vi "CRYGet Next Color.vi"(11 "Type":enum16{"Curves", "Values", "Results", "WFM"}(ring)) -> (3 "Color":u32)   [LabVIEW 2013]
uses:
  Global/CRYCurve Library Global.vi
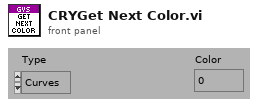
[diagram p1: front panel]
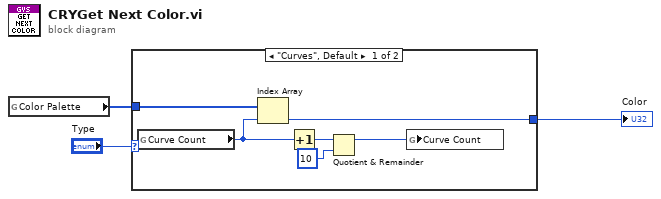
[diagram p0: block diagram]
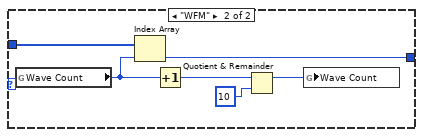
[diagram p2: hidden frame]
diagram:
  n1 = global read "CRYCurve Library Global.vi" "Color Palette"() -> (w2:u32[])
  n2 = case shown="\"Curves\", Default" "Type" {
    tunnel: w2 -> [w9 w15]
    tunnel: [w8 w14] -> w1
    frame "Curves", Default {
      n3 = global read "CRYCurve Library Global.vi" "Curve Count"() -> (w7:i32)
      n4 = Index Array(array=w9, index=w7) -> (element=w8:u32)
      n5 = Increment(x=w7) -> (x+1=w6:i32)
      n6 = Quotient & Remainder(x=w6, y=10) -> (x-y*floor(x/y)=w4:i32)  [unwired: 1 out]
      n7 = global write "CRYCurve Library Global.vi" "Curve Count"(w4) -> ()
    }
    frame "WFM" {
      n8 = global read "CRYCurve Library Global.vi" "Wave Count"() -> (w13:i32)
      n9 = Index Array(array=w15, index=w13) -> (element=w14:u32)
      n10 = Increment(x=w13) -> (x+1=w11:i32)
      n11 = Quotient & Remainder(x=w11, y=10) -> (x-y*floor(x/y)=w10:i32)  [unwired: 1 out]
      n12 = global write "CRYCurve Library Global.vi" "Wave Count"(w10) -> ()
    }
  }
  "Color" <- w1
